vi "Line length bipolar split.vi"(11 "Line length":i32) -> (1 "Positive length":i32, 3 "Negative length":i32)   [LabVIEW 2017]
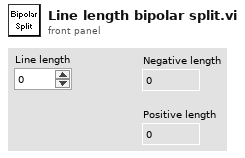
[diagram p1: front panel]
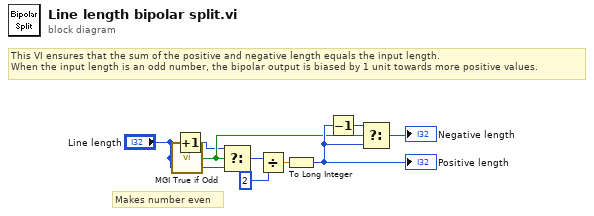
[diagram p0: block diagram]
diagram:
  # "This VI ensures that the sum of the positive and negative length equals the input length.\nWhen the input length is an odd number, the bipolar output is biased by 1 unit towards more positive values."
  # "Makes number even"
  n1 = call <userlib>:"MGI True if Odd.vi"("Integer"="Line length") -> ("Odd?"=w6:bool)
  n2 = Increment(x="Line length") -> (x+1=w3:i32)
  n3 = Select(t=w3, s=w6, f="Line length") -> (s? t:f=w5:i32)
  n4 = Divide(x=w5, y=2) -> (x/y=w2:dbl)
  n5 = To Long Integer(number=w2) -> (32bit integer=w7:i32)
  "Positive length" <- w7
  n6 = Decrement(x=w7) -> (x-1=w8:i32)
  n7 = Select(t=w8, s=w6, f=w7) -> (s? t:f=→"Negative length":i32)
